vi "New Group.vi"(8 "error in (no error)":errorcluster, 11 "BluelinesRedlines in":refnum<class "BluelinesRedlines.lvclass">) -> (0 "error out":errorcluster, 3 "BluelinesRedlines out":refnum<class "BluelinesRedlines.lvclass">)   [LabVIEW 2020, in "VolatusGUIElements.lvlib" / "BluelinesRedlines.lvclass"]
uses:
  BluelinesRedlines.lvclass
  BluelinesRedlines.lvclass/BluelinesRedlines.ctl
  User BluelinesRedlines/User BluelinesRedlines.lvclass
  C:/dev/lv20CE/relink/lv-volatus/VolatusGUIElements/User BluelinesRedlines/User BluelinesRedlines.lvclass
  C:/dev/lv20CE/relink/lv-volatus/VolatusGUI/BluelinesRedlines Source/BluelinesRedlines Source.lvclass
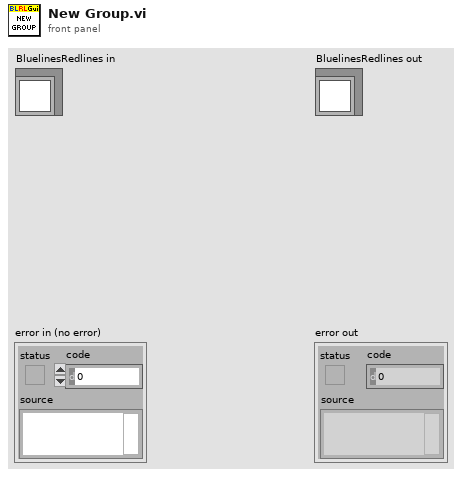
[diagram p1: front panel]
types:
  T1 = map{string, refnum<class "BluelinesRedlines Source.lvclass">}
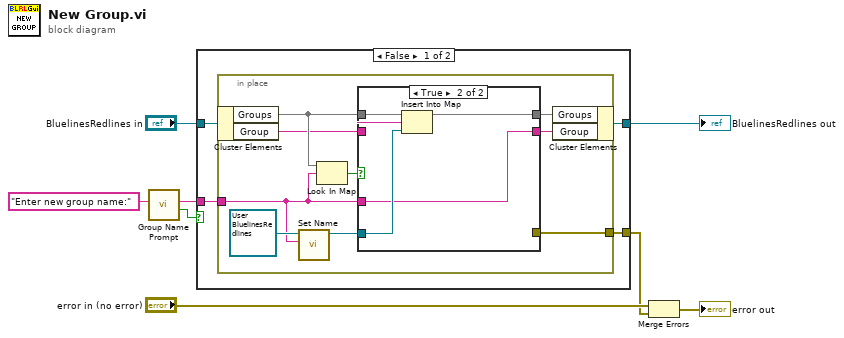
[diagram p0: block diagram]
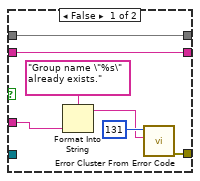
[diagram p2: hidden frame]
diagram:
  n1 = call "Group Name Prompt.vi"("Prompt"="Enter new group name:") -> ("Cancelled"=w5:bool, "Name"=w4:string)  [unwired: 9 in]
  n2 = case shown="False" w5 {
    tunnel: "BluelinesRedlines in" -> [w12 w33]
    tunnel: w4 -> [w11 _]
    tunnel: [w10 w33] -> w3
    tunnel: [w9 _] -> w1
    frame False {
      n3 = in-place {
        in-place-border: w11 -> [w17]
        in-place-border: [w13] -> w9
        n4 = in-place-cluster #1(w12) -> ("Groups"=w18:T1, "Group"=w14:string)
        n5 = call "Set Name.vi"("Name"=w17, "User BluelinesRedlines in"=refnum<class "User BluelinesRedlines.lvclass"> refnum ("VolatusGUIElements.lvlib:User BluelinesRedlines.lvclass")) -> ("User BluelinesRedlines out"=w20:refnum<class "User BluelinesRedlines.lvclass">)  [unwired: 8 in, 1 out]
        n6 = Look In Map(map=w18, key=w17) -> (key not found?=w16:bool)  [unwired: 1 in, 1 out]
        n7 = case shown="True" w16 {
          tunnel: w20 -> [_ w32]
          tunnel: [w27 w31] -> w19
          tunnel: w18 -> [w27 w30]
          tunnel: w17 -> [w24 w29]
          tunnel: [w28 w29] -> w15
          tunnel: w14 -> [w28 _]
          tunnel: [w22 _] -> w13
          frame False {
            n8 = Format Into String(format string="Group name \"%s\" already exists.", w24) -> (resulting string=w23:string)  [unwired: 2 in, 1 out]
            n9 = call <vilib>:"Error Cluster From Error Code.vi"("error message (\"\")"=w23, "error code (0)"=131) -> ("error out"=w22:errorcluster)  [unwired: 7 in]
          }
          frame True {
            n10 = Insert Into Map(map in=w30, key=w29, value=w32) -> (map out=w31:T1)  [unwired: 2 out]
          }
        }
        n11 = in-place-cluster #1("Groups"=w19, "Group"=w15) -> (w10:refnum<class "BluelinesRedlines.lvclass">)
      }
    }
    frame True {
    }
  }
  "BluelinesRedlines out" <- w3
  n12 = Merge Errors("error in (no error)", w1) -> (→"error out":errorcluster)
